vi "Kontaktpositionen_finden.vi"(8 "Fehler in":errorcluster, 10 "Größe Kontaktsuchfeld":sgl=70.0, 11 "Cluster in":T1={"Initialisierung"={"Online?"=FALSE, "Grundpfad"=path "", "Kamera Oben"="", "IP-Adresse Flüssiglinse"="", "Flüssiglinse"=refnum, "Kamera Unten"="", "IP-Adresse SPS"="", "SPS-Verbindung"={"TCP Connection Ref"=refnum, "IP address"="", "timeout ms"=5000, "Connected?"=FALSE, "PLC Type"=enum."S7 1200", "Rack S7 400"=0, "Slot S7 400"=0, "PDU Size"=0, "connection semaphore"=refnum}, "IP-Adresse Lichtgitter"="", "Lichtgitter"=refnum, "Skalierungsfaktor"=0.0, "Bilder Oben"=[], "Bild Unten"=refnum, "Bild Ausschnitt Unten"=refnum}, "Einstellungen"={"Gesamtablauf gestartet"=FALSE, "i. O. Bilder speichern"=FALSE, "Bildspeicherung Offline"=FALSE, "Ausgewähltes Offline-Datum"="", "Ausgewähltes Offline-Teil"="", "Speicherpfad Bilder"=path ""}, "Artikeldaten"={"Artikelnummer"="", "Fertigungsauftrag"="", "Muster ISO"=refnum, "Belichtungszeit Referenzmarken"=0.0, "Fokus Referenzmarken"=0.0, "Belichtungszeit ISO"=0.0, "Fokus ISO"=0.0, "Belichtungszeit Unten"=0.0, "Kontaktanzahl"=0, "Aktueller Kontakt"=0, "Kontaktposition"={"x"=0.0, "y"=0.0}, "ISO-Muster nicht vorhanden"=FALSE, "Winkel ISO"=0.0, "Mittelpunkt ISO"={"x"=0.0, "y"=0.0}}, "Werte Kamera Oben"={"Koordinatensystem"={"Punkt x-Achse"={"X"=0.0, "Y"=0.0}, "Ursprung"={"X"=0.0, "Y"=0.0}, "Punkt y-Achse"={"X"=0.0, "Y"=0.0}}, "Position Kontakt"={"x"=0.0, "y"=0.0}, "Durchmesser Loch"=0.0, "Winkel Kontakt"=0.0}, "Werte Kamera Unten"={"Prüfung Unten n. i. O."=FALSE}, "Werte Lichtgitter"={"Messwerte Referenzmarken"=[], "Mittelpunkt Referenzmarken"={"x"=0.0, "y"=0.0}, "Messwerte Kontakt"=[], "Offset"={"x"=0.0, "y"=0.0}}, "Rückmeldungen"={"Koordinaten ermittelt"=FALSE, "Vermessung Lichtgitter fertig"=FALSE, "Nachkontrolle Kamera Unten fertig"=FALSE}, "Fehler"={"Referenzen nicht gefunden"=FALSE, "Kontakt nicht gefunden"=FALSE, "Referenzen nicht in Lichtgitter"=FALSE, "Kontakt zu groß"=FALSE, "Kontakt zu klein"=FALSE}, "Statistik"={"Statistiken"=[]}, "Timer"={"Timer Start Position"=0, "Timer Start Lichtgitter"=0, "Timer Start Kamera Unten"=0}}) -> (0 "Fehler out":errorcluster, 2 "Kontakt nicht gefunden":bool, 3 "Cluster out":T1={"Initialisierung"={"Online?"=FALSE, "Grundpfad"=path "", "Kamera Oben"="", "IP-Adresse Flüssiglinse"="", "Flüssiglinse"=refnum, "Kamera Unten"="", "IP-Adresse SPS"="", "SPS-Verbindung"={"TCP Connection Ref"=refnum, "IP address"="", "timeout ms"=5000, "Connected?"=FALSE, "PLC Type"=enum."S7 1200", "Rack S7 400"=0, "Slot S7 400"=0, "PDU Size"=0, "connection semaphore"=refnum}, "IP-Adresse Lichtgitter"="", "Lichtgitter"=refnum, "Skalierungsfaktor"=0.0, "Bilder Oben"=[], "Bild Unten"=refnum, "Bild Ausschnitt Unten"=refnum}, "Einstellungen"={"Gesamtablauf gestartet"=FALSE, "i. O. Bilder speichern"=FALSE, "Bildspeicherung Offline"=FALSE, "Ausgewähltes Offline-Datum"="", "Ausgewähltes Offline-Teil"="", "Speicherpfad Bilder"=path ""}, "Artikeldaten"={"Artikelnummer"="", "Fertigungsauftrag"="", "Muster ISO"=refnum, "Belichtungszeit Referenzmarken"=0.0, "Fokus Referenzmarken"=0.0, "Belichtungszeit ISO"=0.0, "Fokus ISO"=0.0, "Belichtungszeit Unten"=0.0, "Kontaktanzahl"=0, "Aktueller Kontakt"=0, "Kontaktposition"={"x"=0.0, "y"=0.0}, "ISO-Muster nicht vorhanden"=FALSE, "Winkel ISO"=0.0, "Mittelpunkt ISO"={"x"=0.0, "y"=0.0}}, "Werte Kamera Oben"={"Koordinatensystem"={"Punkt x-Achse"={"X"=0.0, "Y"=0.0}, "Ursprung"={"X"=0.0, "Y"=0.0}, "Punkt y-Achse"={"X"=0.0, "Y"=0.0}}, "Position Kontakt"={"x"=0.0, "y"=0.0}, "Durchmesser Loch"=0.0, "Winkel Kontakt"=0.0}, "Werte Kamera Unten"={"Prüfung Unten n. i. O."=FALSE}, "Werte Lichtgitter"={"Messwerte Referenzmarken"=[], "Mittelpunkt Referenzmarken"={"x"=0.0, "y"=0.0}, "Messwerte Kontakt"=[], "Offset"={"x"=0.0, "y"=0.0}}, "Rückmeldungen"={"Koordinaten ermittelt"=FALSE, "Vermessung Lichtgitter fertig"=FALSE, "Nachkontrolle Kamera Unten fertig"=FALSE}, "Fehler"={"Referenzen nicht gefunden"=FALSE, "Kontakt nicht gefunden"=FALSE, "Referenzen nicht in Lichtgitter"=FALSE, "Kontakt zu groß"=FALSE, "Kontakt zu klein"=FALSE}, "Statistik"={"Statistiken"=[]}, "Timer"={"Timer Start Position"=0, "Timer Start Lichtgitter"=0, "Timer Start Kamera Unten"=0}})   [LabVIEW 2024]
uses:
  Typdefinitionen/Cluster.ctl
  <vilib>/userDefined/High Color/IMAQdx.ctl
  <vilib>/DATA AHEAD/SP7/typedefs/S7 Connection.ctl
  <vilib>/DATA AHEAD/SP7/typedefs/PLC Type.ctl
  <vilib>/vision/Image Controls.llb/IMAQ Image.ctl
  Typdefinitionen/Koordinatensystem.ctl
  Typdefinitionen/Statistik.ctl
  <vilib>/vision/Pattern Matching.llb/IMAQ Curve Parameters.ctl
  <vilib>/vision/NI_Vision_Development_Module.lvlib
  <vilib>/DATA AHEAD/SP7/SP7.lvlib
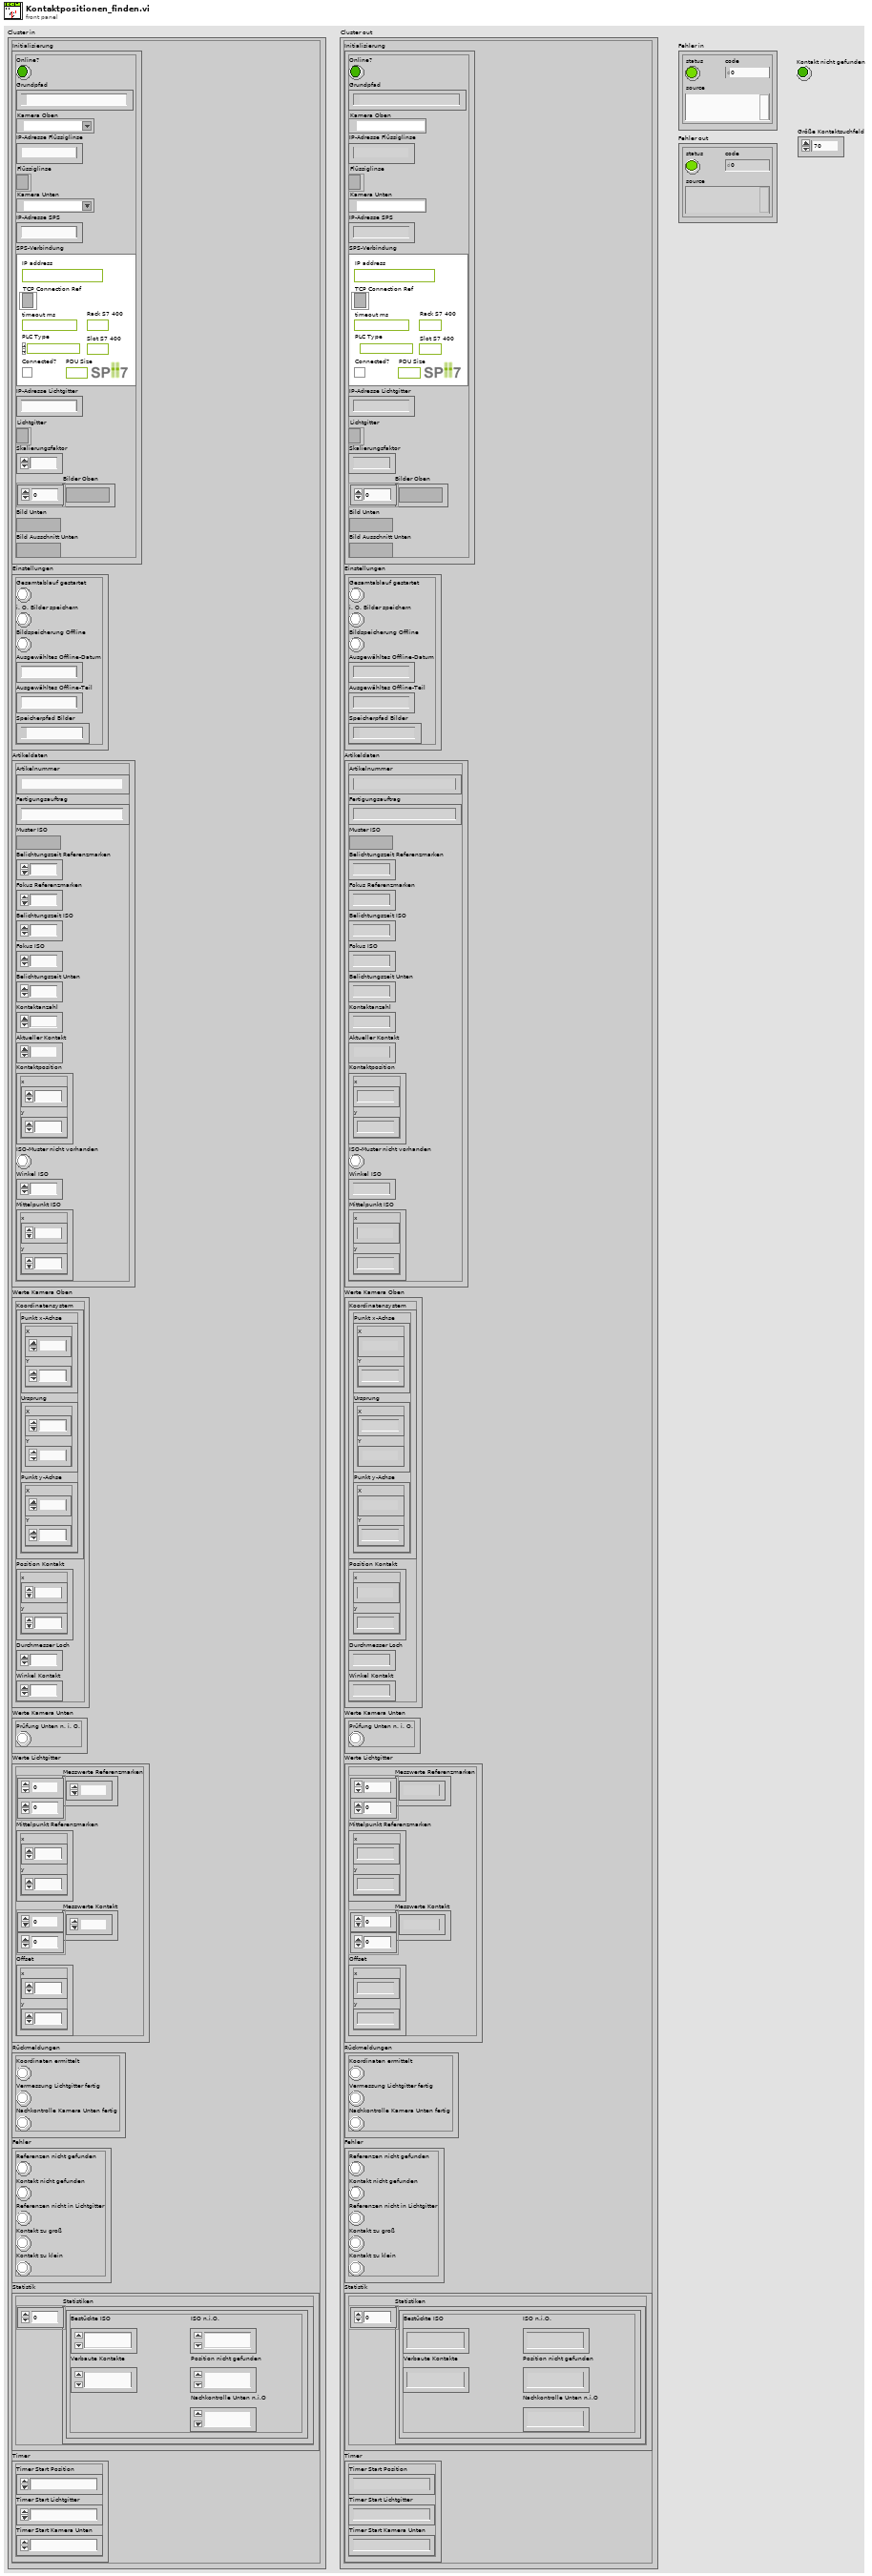
[diagram p1: front panel]
types:
  T1 = typedef "Cluster.ctl" = cluster{"Initialisierung":cluster{"Online?":bool, "Grundpfad":path, "Kamera Oben":T2, "IP-Adresse Flüssiglinse":string, "Flüssiglinse":refnum<k5>, "Kamera Unten":T2, "IP-Adresse SPS":string, "SPS-Verbindung":T3, "IP-Adresse Lichtgitter":string, "Lichtgitter":refnum<k5>, "Skalierungsfaktor":dbl, "Bilder Oben":T6[], "Bild Unten":T6, "Bild Ausschnitt Unten":T6}, "Einstellungen":cluster{"Gesamtablauf gestartet":bool, "i. O. Bilder speichern":bool, "Bildspeicherung Offline":bool, "Ausgewähltes Offline-Datum":string, "Ausgewähltes Offline-Teil":string, "Speicherpfad Bilder":path}, "Artikeldaten":cluster{"Artikelnummer":string, "Fertigungsauftrag":string, "Muster ISO":T6, "Belichtungszeit Referenzmarken":dbl, "Fokus Referenzmarken":dbl, "Belichtungszeit ISO":dbl, "Fokus ISO":dbl, "Belichtungszeit Unten":dbl, "Kontaktanzahl":u32, "Aktueller Kontakt":i16, "Kontaktposition":cluster{"x":sgl, "y":sgl}, "ISO-Muster nicht vorhanden":bool, "Winkel ISO":sgl, "Mittelpunkt ISO":cluster{"x":dbl, "y":dbl}}, "Werte Kamera Oben":cluster{"Koordinatensystem":T7, "Position Kontakt":cluster{"x":dbl, "y":dbl}, "Durchmesser Loch":dbl, "Winkel Kontakt":dbl}, "Werte Kamera Unten":cluster{"Prüfung Unten n. i. O.":bool}, "Werte Lichtgitter":cluster{"Messwerte Referenzmarken":dbl[][], "Mittelpunkt Referenzmarken":cluster{"x":dbl, "y":dbl}, "Messwerte Kontakt":dbl[][], "Offset":cluster{"x":dbl, "y":dbl}}, "Rückmeldungen":cluster{"Koordinaten ermittelt":bool, "Vermessung Lichtgitter fertig":bool, "Nachkontrolle Kamera Unten fertig":bool}, "Fehler":cluster{"Referenzen nicht gefunden":bool, "Kontakt nicht gefunden":bool, "Referenzen nicht in Lichtgitter":bool, "Kontakt zu groß":bool, "Kontakt zu klein":bool}, "Statistik":cluster{"Statistiken":T8[]}, "Timer":cluster{"Timer Start Position":u32, "Timer Start Lichtgitter":u32, "Timer Start Kamera Unten":u32}}
  T2 = typedef "IMAQdx.ctl" = refnum<k21>
  T3 = typedef "SP7.lvlib/S7 Connection.ctl" = cluster{"TCP Connection Ref":refnum<k5>, "IP address":string, "timeout ms":i32, "Connected?":bool, "PLC Type":T4, "Rack S7 400":u8, "Slot S7 400":u8, "PDU Size":u16, "connection semaphore":T5}
  T4 = typedef "SP7.lvlib/PLC Type.ctl" = enum16{"S7 200", "S7 300/400", "S7 1200", "S7 1500", "LOGO!8"}
  T5 = typedef "Semaphore RefNum" = refnum<k1>
  T6 = typedef "IMAQ Image.ctl" = refnum<image>
  T7 = typedef "Koordinatensystem.ctl" = cluster{"Punkt x-Achse":cluster{"X":sgl, "Y":sgl}, "Ursprung":cluster{"X":sgl, "Y":sgl}, "Punkt y-Achse":cluster{"X":sgl, "Y":sgl}}
  T8 = typedef "Statistik.ctl" = cluster{"Bestückte ISO":u32, "Verbaute Kontakte":u32, "ISO n.i.O.":u32, "Nachkontrolle Unten n.i.O":u32, "Position nicht gefunden":u32}
  T9 = typedef "IMAQ Curve Parameters.ctl" = cluster{"Extraction Mode":u32, "Edge Threshold":i32, "Edge Filter Size":u32, "Min Length":i32, "Row Search Step Size":i32, "Col Search Step Size":i32, "Max Endpoint Gap":i32, "Closed":bool, "Subpixel":bool}
  T10 = typedef "IMAQ Rectangle" = cluster{"Left":i32, "Top":i32, "Right":i32, "Bottom":i32, "Rotation":dbl}
  T11 = typedef "ROI Descriptor" = cluster{"Global Rectangle":i32[], "Contours":cluster{"ID":enum32{"External", "Internal"}, "Type":u32, "Coordinates":i32[]}[]}
  T12 = cluster{"Position":cluster{"X":sgl, "Y":sgl}, "Radius":dbl, "Score":dbl}[]
  T13 = cluster{"Farbe Kreis":u32, "Kreis ausfüllen?":bool, "Bounding Rechteck anzeigen?":bool, "Farbe Bounding Rechteck":u32}
  T14 = cluster{"Position":cluster{"X":sgl, "Y":sgl}, "Radius":dbl, "Score":dbl}
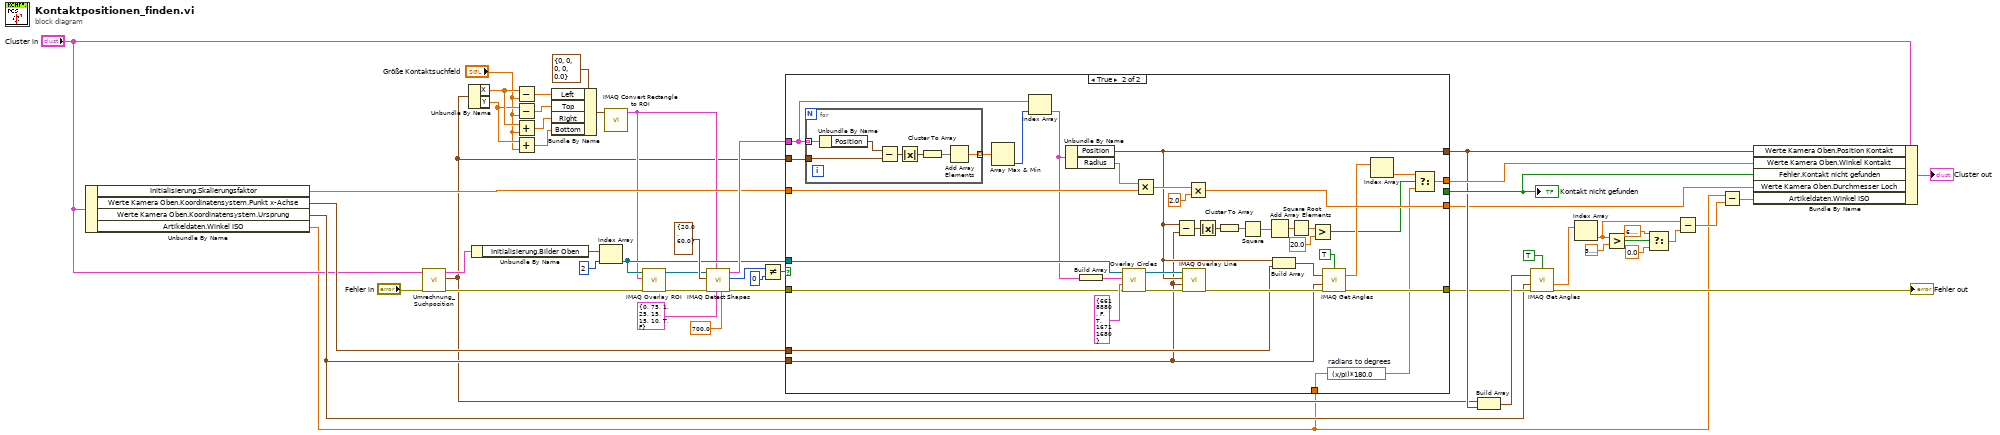
[diagram p0: block diagram]
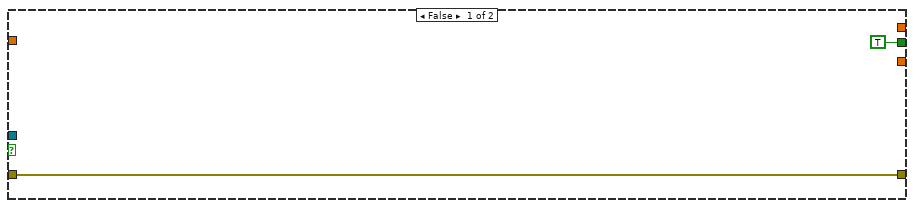
[diagram p2: hidden frame]
diagram:
  n1 = Unbundle By Name("Cluster in") -> ("Initialisierung.Skalierungsfaktor"=w30:dbl, "Werte Kamera Oben.Koordinatensystem.Punkt x-Achse"=w29:cluster{"X":sgl, "Y":sgl}, "Werte Kamera Oben.Koordinatensystem.Ursprung"=w9:cluster{"X":sgl, "Y":sgl}, "Artikeldaten.Winkel ISO"=w1:sgl)
  n2 = call "Umrechnung_Suchposition.vi"("error in"="Fehler in", "Cluster in"="Cluster in") -> ("error out"=w4:errorcluster, "Koordinaten out"=w2:cluster{"X":sgl, "Y":sgl}, "Cluster out"=w3:T1)  [unwired: 7 in]
  n3 = Unbundle By Name(w2) -> ("X"=w43:sgl, "Y"=w42:sgl)
  n4 = Unbundle By Name(w3) -> ("Initialisierung.Bilder Oben"=w48:T6[])
  n5 = Subtract(x=w43, y="Größe Kontaktsuchfeld") -> (x-y=w44:sgl)
  n6 = Subtract(x=w42, y="Größe Kontaktsuchfeld") -> (x-y=w41:sgl)
  n7 = Add(x=w43, y="Größe Kontaktsuchfeld") -> (x+y=w40:sgl)
  n8 = Add(x=w42, y="Größe Kontaktsuchfeld") -> (x+y=w39:sgl)
  n9 = Bundle By Name(cluster=T10 {"Left"=0, "Top"=0, "Right"=0, "Bottom"=0, "Rotation"=0.0} ("Rectangle"), "Left"=w44, "Top"=w41, "Right"=w40, "Bottom"=w39) -> (w45:T10)
  n10 = Index Array(array=w48, index=2 ("t")) -> (element=w27:T6)
  n11 = call "IMAQ Convert Rectangle to ROI"("Rectangle"=w45) -> ("ROI Descriptor"=w26:T11)  [unwired: 8 in, 1 out]
  n12 = call "IMAQ Overlay ROI"("error in (no error)"=w4, "ROI Descriptor"=w26, "Image"=w27) -> ("error out"=w38:errorcluster, "Image Out"=w37:T6)  [unwired: 7 in]
  n13 = call-poly "IMAQ Detect Shapes"("Minimum match score"=700.0, "Curve Parameters"=T9 {"Extraction Mode"=0, "Edge Threshold"=75, "Edge Filter Size"=1, "Min Length"=25, "Row Search Step Size"=15, "Col Search Step Size"=15, "Max Endpoint Gap"=10, "Closed"=TRUE, "Subpixel"=FALSE}, "ROI Descriptor"=w26, "error in (no error)"=w38, "Circle Descriptor"=cluster{"Min Radius":dbl, "Max Radius":dbl} {"Min Radius"=20.0, "Max Radius"=60.0}, "Image"=w37) -> ("error out"=w36:errorcluster, "Number of Matches Returned"=w24:i32, "Circles"=w35:T12)  [unwired: 3 in]
  n14 = Not Equal?(x=w24, y=0) -> (x != y?=w33:bool)
  n15 = case shown="True" w33 {
    tunnel: [w52 w75] -> w11
    tunnel: [_ w70] -> w21
    tunnel: w9 -> [_ w69]
    tunnel: w30 -> [_ w83]
    tunnel: [_ w80] -> w7
    tunnel: w27 -> [_ w79]
    tunnel: w36 -> [w52 w78]
    tunnel: w35 -> [_ w55]
    tunnel: [TRUE ("Kontakt nicht gefunden") _] -> w23
    tunnel: w29 -> [_ w73]
    tunnel: [_ w60] -> w28
    tunnel: w2 -> [_ w57]
    tunnel: w1 -> [_ w53]
    frame False {
    }
    frame True {
      n16 = for {
        tunnel: w55 -> [w95] mode=indexing
        tunnel: w57 -> [w92]
        tunnel: [w89] -> w56 mode=indexing
        n17 = Unbundle By Name(w95) -> ("Position"=w93:cluster{"X":sgl, "Y":sgl})
        n18 = Subtract(x=w93, y=w92) -> (x-y=w94:cluster{"X":sgl, "Y":sgl})
        n19 = Absolute Value(x=w94) -> (abs(x)=w91:cluster{"X":sgl, "Y":sgl})
        n20 = Cluster To Array(cluster=w91) -> (array=w90:sgl[])
        n21 = Add Array Elements(numeric array=w90) -> (sum=w89:sgl)
      }
      n22 = Array Max & Min(array=w56) -> (min index (indices)=w54:i32)  [unwired: 3 out]
      n23 = Index Array(array=w55, index=w54) -> (element=w58:T14)
      n24 = Unbundle By Name(w58) -> ("Position"=w70:cluster{"X":sgl, "Y":sgl}, "Radius"=w84:dbl)
      n25 = Build Array(w58) -> (w88:T12)
      n26 = call "Overlay Circles.vi"("error in"=w78, "Einstellungen"=T13 {"Farbe Kreis"=6618880, "Kreis ausfüllen?"=FALSE, "Bounding Rechteck anzeigen?"=TRUE, "Farbe Bounding Rechteck"=16711680}, "Circles"=w88, "Image in"=w79) -> ("error out"=w86:errorcluster, "Image out"=w85:T6)  [unwired: 6 in]
      n27 = Multiply(x=w84, y=w83) -> (x*y=w82:dbl)
      n28 = Subtract(x=w70, y=w69) -> (x-y=w71:cluster{"X":sgl, "Y":sgl})
      n29 = call "IMAQ Overlay Line"("error in (no error)"=w86, "End Point"=w69, "Start Point"=w70, "Image"=w85) -> ("error out"=w76:errorcluster)  [unwired: 6 in, 1 out]
      n30 = Multiply(x=w82, y=2.0) -> (x*y=w80:dbl)
      n31 = Absolute Value(x=w71) -> (abs(x)=w68:cluster{"X":sgl, "Y":sgl})
      n32 = Cluster To Array(cluster=w68) -> (array=w66:sgl[])
      n33 = Square(x=w66) -> (x^2=w67:sgl[])
      n34 = Add Array Elements(numeric array=w67) -> (sum=w65:sgl)
      n35 = Build Array(w70, w73) -> (w74:cluster{"X":sgl, "Y":sgl}[])
      n36 = Square Root(x=w65) -> (sqrt(x)=w64:sgl)
      n37 = Greater?(x=w64, y=sgl 20.0) -> (0:w62:bool)
      n38 = call "IMAQ Get Angles"("error in (no error)"=w76, "Vertex"=w69, "Points"=w74, "Use Vertex (No)"=TRUE) -> ("error out"=w75:errorcluster, "Angles (deg)"=w72:sgl[])  [unwired: 1 in, 1 out]
      n39 = expression code="(x/pi)*180.0" "radians to degrees"(w53) -> (w59:sgl)
      n40 = Index Array(array=w72) -> (element=w61:sgl)  [unwired: 1 in]
      n41 = Select(t=w61, s=w62, f=w59) -> (s? t:f=w60:sgl)
    }
  }
  "Kontakt nicht gefunden" <- w23
  n42 = Build Array(w2, w21) -> (w20:cluster{"X":sgl, "Y":sgl}[])
  n43 = call "IMAQ Get Angles"("error in (no error)"=w11, "Vertex"=w9, "Points"=w20, "Use Vertex (No)"=TRUE) -> ("error out"=→"Fehler out":errorcluster, "Angles (rad)"=w19:sgl[])  [unwired: 1 in, 1 out]
  n44 = Index Array(array=w19) -> (element=w14:sgl)  [unwired: 1 in]
  n45 = Greater?(x=w14, y=3.141592653589793) -> (0:w17:bool)
  n46 = Select(t=6.283185307179586, s=w17, f=0.0) -> (s? t:f=w13:dbl)
  n47 = Subtract(x=w14, y=w13) -> (x-y=w12:dbl)
  n48 = Subtract(x=w1, y=w12) -> (x-y=w8:dbl)
  n49 = Bundle By Name(cluster="Cluster in", "Werte Kamera Oben.Position Kontakt"=w21, "Werte Kamera Oben.Winkel Kontakt"=w28, "Fehler.Kontakt nicht gefunden"=w23, "Werte Kamera Oben.Durchmesser Loch"=w7, "Artikeldaten.Winkel ISO"=w8) -> (→"Cluster out":T1)
